vi "Connect.vi"(8 "error in (no error)":errorcluster, 11 "Yokogawa AQ6370D in":refnum<class "Yokogawa AQ6370D.lvclass">) -> (0 "error out":errorcluster, 3 "Yokogawa AQ6370D out":refnum<class "Yokogawa AQ6370D.lvclass">)   [LabVIEW 2018, in "Yokogawa AQ6370D.lvlib" / "Yokogawa AQ6370D.lvclass"]
uses:
  Yokogawa AQ6370D.lvclass
  Yokogawa AQ6370D.lvclass/Yokogawa AQ6370D.ctl
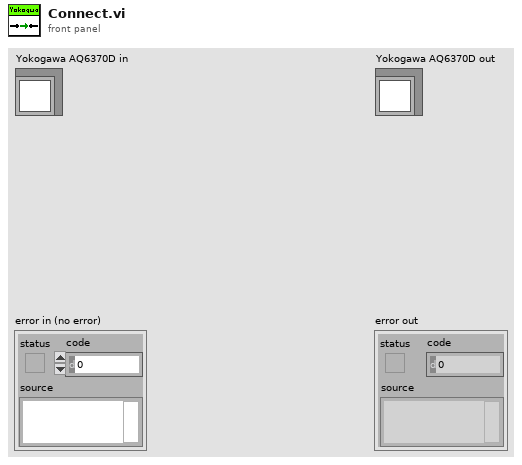
[diagram p1: front panel]
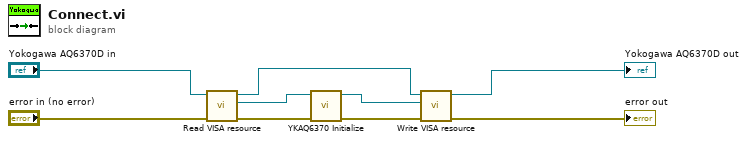
[diagram p0: block diagram]
diagram:
  n1 = call "Read VISA resource.vi"("error in (no error)"="error in (no error)", "Yokogawa AQ6370D in"="Yokogawa AQ6370D in") -> ("error out"=w7:errorcluster, "VISA resource"=w2:refnum<visa-resource-name>, "Yokogawa AQ6370D out"=w4:refnum<class "Yokogawa AQ6370D.lvclass">)  [unwired: 7 in]
  n2 = call <instrlib>:"YKAQ6370 Initialize.vi"("error in (no error)"=w7, "VISA resource name"=w2) -> ("error out"=w6:errorcluster, "VISA resource name out"=w3:refnum<visa-resource-name>)  [unwired: 8 in]
  n3 = call "Write VISA resource.vi"("error in (no error)"=w6, "VISA resource"=w3, "Yokogawa AQ6370D in"=w4) -> ("error out"=→"error out":errorcluster, "Yokogawa AQ6370D out"=→"Yokogawa AQ6370D out":refnum<class "Yokogawa AQ6370D.lvclass">)  [unwired: 7 in]
